vi "isDone.vi"(8 "error in (no error)":errorcluster, 11 "GuassianNoiseWave in":refnum<class "GuassianNoiseWave.lvclass">) -> (0 "error out":errorcluster, 2 "isDone?":bool=TRUE, 3 "GuassianNoiseWave out":refnum<class "GuassianNoiseWave.lvclass">)   [LabVIEW 2015, in "GuassianNoiseWave.lvclass"]
uses:
  GuassianNoiseWave.lvclass
  GuassianNoiseWave.lvclass/GuassianNoiseWave.ctl
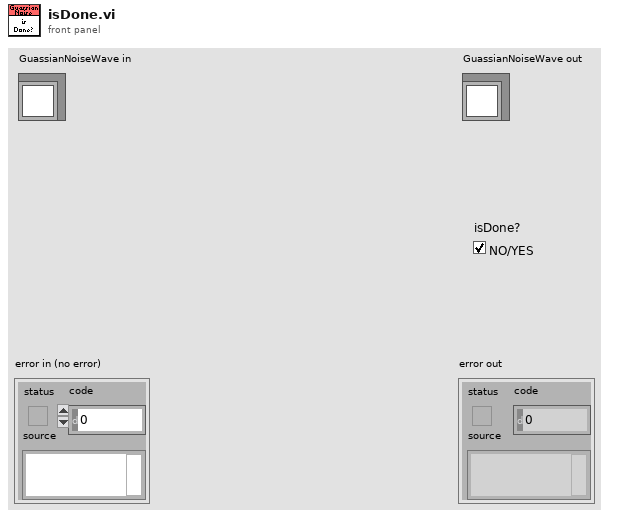
[diagram p1: front panel]
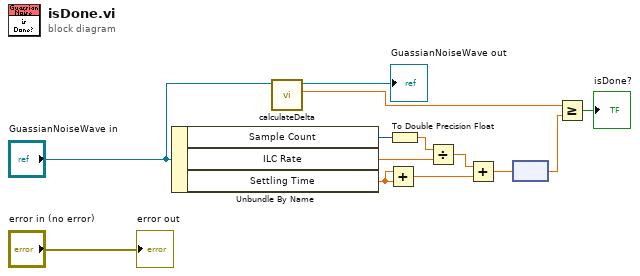
[diagram p0: block diagram]
diagram:
  n1 = Unbundle By Name("GuassianNoiseWave in") -> ("Sample Count"=w9:u32, "ILC Rate"=w8:dbl[unit], "Settling Time"=w7:dbl[unit])
  n2 = call "calculateDelta.vi"("GuassianNoiseWave in"="GuassianNoiseWave in") -> ("Delta Timestamp"=w3:dbl, "GuassianNoiseWave out"=→"GuassianNoiseWave out":refnum<class "GuassianNoiseWave.lvclass">)  [unwired: 8 in, 1 out]
  n3 = Add(x=w7, y=w7) -> (x+y=w10:dbl[unit])
  n4 = To Double Precision Float(number=w9) -> (double precision float=w12:dbl)
  n5 = Divide(x=w12, y=w8) -> (x/y=w11:dbl[unit])
  n6 = Add(x=w11, y=w10) -> (x+y=w5:dbl[unit])
  n7 = node(w5) -> (w6:dbl)
  n8 = Greater Or Equal?(x=w3, y=w6) -> (x >= y?=→"isDone?":bool)
  "error out" <- "error in (no error)"
